vi "MagnetoCaloricSweep_wendel.vi"(9 "Measure for (s)":dbl=5.0, 11 "UseCommandLine":bool=TRUE) -> (1 "Sample temperatur":dbl[](array[numeric]), 2 "Bath Temperature":dbl[](array[numeric]), 3 "Time":u32[](array[numeric]), 4 "XY Graph":cluster{dbl[], dbl[]}[](graph))   [LabVIEW 2019]
uses:
  Instrument_Setup.vi
  Global/Global Variables/Data_Display_global.vi
  Equipment/Lake Shore 372/Lake Shore 372.lvlib
panel:
  in  "Additional LS370":refnum<visa-resource-name>="GPIB0::18::INSTR"
  out "Wait":bool
  in  "Dateipfad (Dialog verwenden)":path
  out "Phi":dbl[](array[numeric])
  out "Field":dbl[](array[numeric])
  out "Indices":i32[](array[numeric])
  out "R2":dbl
  out "R1":dbl
  out "T2":dbl
  out "T1":dbl
  out "Phi":dbl
  out "B":dbl
  in  "StopSkript":bool
  # "current values"
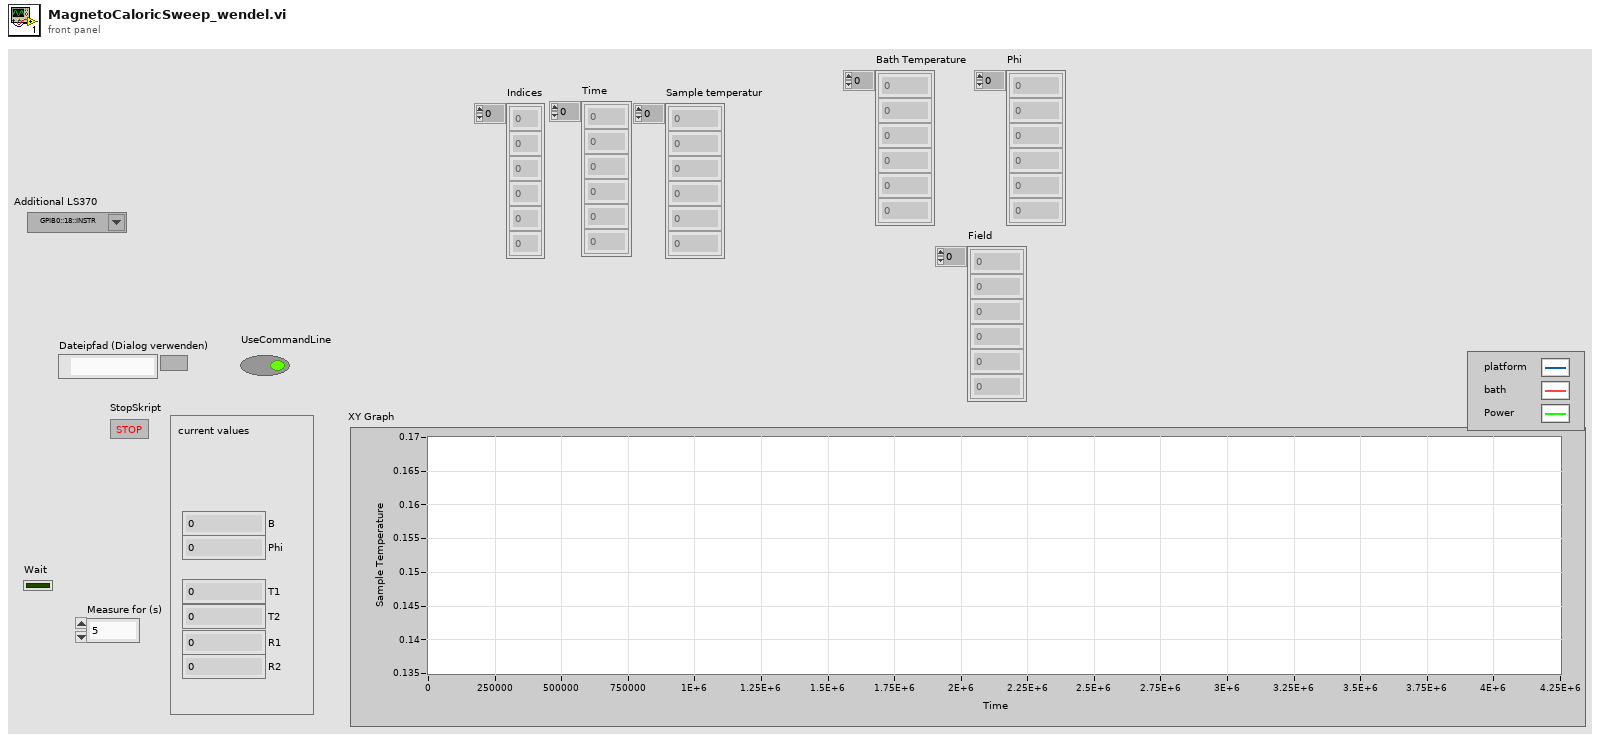
[diagram p1: front panel]
types:
  T1 = enum16{"open", "replace", "create", "open or create", "replace or create", "replace or create with confirmation"}
  T2 = typedef "AMI_cluster.ctl" = cluster{"Y Axis Status":enum16{"", "RAMPING", "HOLDING", "PAUSED", "MANUAL UP", "MANUAL DOWN", "ZEROING CURRENT", "QUENCH DETECTED", "HEATING SWITCH", "AT ZER0", "COOLING SWITCH"}, "Z Axis Status":enum16{"", "RAMPING", "HOLDING", "PAUSED", "MANUAL UP", "MANUAL DOWN", "ZEROING CURRENT", "QUENCH DETECTED", "HEATING SWITCH", "AT ZER0", "COOLING SWITCH"}, "Y-Axis (T)":dbl, "Y-Axis Setpoint (T)":dbl, "Y-Axis Rate (T/min)":dbl, "Z-Axis (T)":dbl, "Z-Axis Setpoint (T)":dbl, "Z-Axis Rate (T/min)":dbl, "B AMI rate (T)":dbl, "AMI Monitor":bool, "AMI Set field rates":bool, "AMI Set field":bool, "Switch Heater Y":bool, "Switch Heater Z":bool, "Switch Heater":bool, "B AMI (T)":dbl, "B AMI Setpoint (T)":dbl, "Phi AMI (Deg) ":dbl, "Phi AMI Setpoint (Deg) ":dbl}
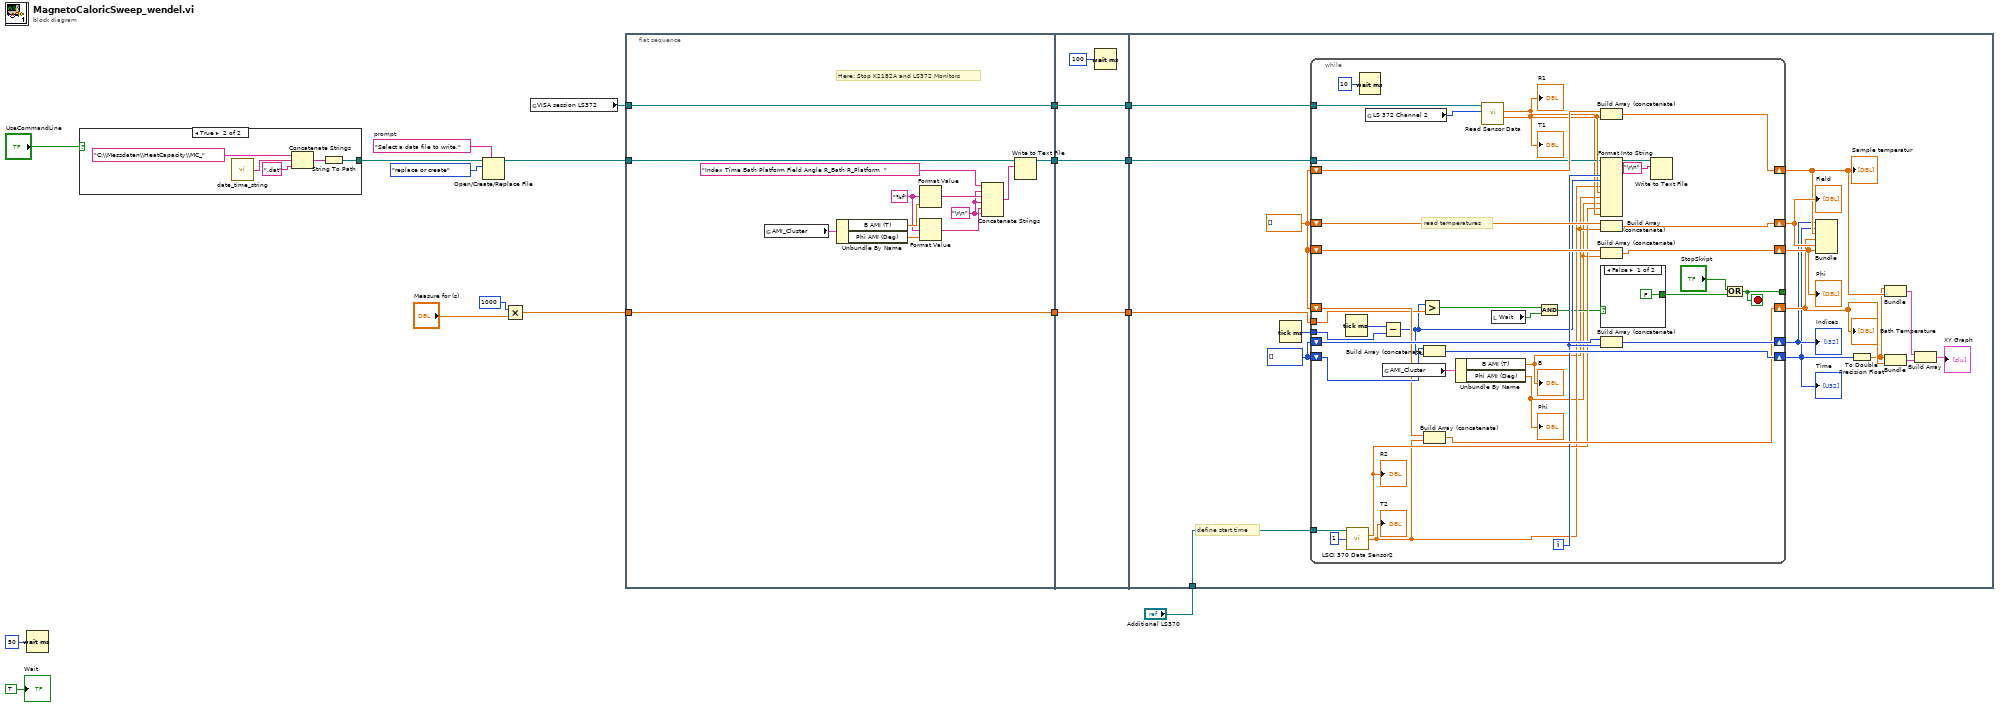
[diagram p0: block diagram]
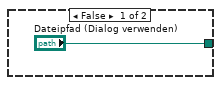
[diagram p2: hidden frame]
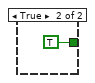
[diagram p3: hidden frame]
diagram:
  w11 = "Select a data file to write."  # prompt
  n1 = Wait (ms)(milliseconds to wait=50) -> ()  [unwired: 1 out]
  n2 = case shown="True" "UseCommandLine" {
    tunnel: ["Dateipfad (Dialog verwenden)" w22] -> w9
    frame False {
    }
    frame True {
      n3 = call "date_time_string.vi"() -> ("date/time string"=w20:string)  [unwired: 1 in]
      n4 = Concatenate Strings("C:\\Messdaten\\HeatCapacity\\MC_", w20, ".dat") -> (w24:string)
      n5 = String To Path(string=w24) -> (path=w22:path)
    }
  }
  n6 = Open/Create/Replace File(file path (use dialog)=w9, prompt=w11, operation (0:open)=T1."replace or create") -> (refnum out=w8:refnum<file>)  [unwired: 3 in, 2 out]
  n7 = Multiply(x=1000, y="Measure for (s)") -> (x*y=w13:dbl)
  n8 = global read "Instrument_Setup.vi" "VISA session LS372"() -> (w17:refnum<visa-resource-name>)
  n9 = flat-sequence {
    tunnel: w13 -> [w36]
    tunnel: w17 -> [w37]
    tunnel: [w37] -> w7
    tunnel: [w36] -> w5
    tunnel: w8 -> [w35]
    tunnel: [w34] -> w3
    tunnel: w7 -> [w41]
    tunnel: [w41] -> w6
    tunnel: w5 -> [w40]
    tunnel: [w40] -> w4
    tunnel: w3 -> [w39]
    tunnel: [w39] -> w2
    tunnel: w6 -> [w58]
    tunnel: w4 -> [w57]
    tunnel: w2 -> [w47]
    tunnel: "Additional LS370" -> [w42]
    frame #0 {
      w27 = "%f"
      w25 = "\r\n"
      # "Here: Stop K2182A and LS372 Monitors"
      n10 = global read "Data_Display_global.vi" "AMI_Cluster"() -> (w31:T2)
      n11 = Unbundle By Name(w31) -> ("B AMI (T)"=w29:dbl, "Phi AMI (Deg)"=w28:dbl)
      n12 = Format Value(format string=w27, value (0)=w29) -> (output string=w30:string)  [unwired: 1 in]
      n13 = Format Value(format string=w27, value (0)=w28) -> (output string=w26:string)  [unwired: 1 in]
      n14 = Concatenate Strings("Index Time Bath Platform Field Angle R_Bath R_Platform  ", w25, w30, w25, w26, w25) -> (w32:string)
      n15 = Write to Text File(file (use dialog)=w35, text=w32) -> (refnum out=w34:refnum<file>)  [unwired: 2 in, 2 out]
    }
    frame #1 {
      n16 = Wait (ms)(milliseconds to wait=100) -> ()  [unwired: 1 out]
    }
    frame #2 {
      w56 = i32[] []
      w55 = dbl[] []
      # "define start time"
      n17 = Tick Count (ms)() -> (millisecond timer value=w46:u32)
      n18 = while {
        shift-right: [w89] -> w45
        shift-left: w56 -> [w90]
        shift-right: [w96] -> w50
        shift-left: w55 -> [w95]
        tunnel: [w75] -> _
        shift-right: [w91] -> w43
        shift-left: w56 -> [w93]
        tunnel: w46 -> [w92]
        tunnel: w58 -> [w67]
        shift-right: [w86] -> w48
        shift-left: w55 -> [w87]
        shift-right: [w84] -> w54
        shift-left: w55 -> [w85]
        shift-right: [w82] -> w53
        shift-left: w55 -> [w83]
        tunnel: w57 -> [w77]
        tunnel: w47 -> [w69]
        tunnel: w42 -> [w63]
        i -> [w81]
        stop <- w75 stop-if-true
        # "read temperatures"
        n19 = Tick Count (ms)() -> (millisecond timer value=w94:u32)
        n20 = call "LSCI 370 Data Sensor2.vi"("VISA session"=w63, "Channel (1)"=1) -> ("Resistance Reading"=w66:dbl, "Kelvin Reading"=w65:dbl)  [unwired: 9 in, 3 out]
        "T2" <- w65
        "R2" <- w66
        n21 = Wait (ms)(milliseconds to wait=10) -> ()  [unwired: 1 out]
        n22 = global read "Instrument_Setup.vi" "LS 372 Channel 2"() -> (w88:u16)
        n23 = Subtract(x=w94, y=w92) -> (x-y=w72:u32)
        n24 = global read "Data_Display_global.vi" "AMI_Cluster"() -> (w62:T2)
        n25 = Greater?(x=w72, y=w77) -> (0:w74:bool)
        n26 = Build Array (concatenate)(w93, w72) -> (w91:u32[])
        n27 = Build Array (concatenate)(w87, w65) -> (w86:dbl[])
        n28 = Unbundle By Name(w62) -> ("B AMI (T)"=w60:dbl, "Phi AMI (Deg)"=w59:dbl)
        "B" <- w60
        "Phi" <- w59
        n29 = call "Read Sensor Data.vi"("Channel (1:1)"=w88, "VISA resource name"=w67) -> ("Kelvin Reading"=w70:dbl, "Resistance Reading"=w68:dbl)  [unwired: 4 in, 4 out]
        "T1" <- w70
        "R1" <- w68
        n30 = local read "Wait"() -> (w73:bool)
        n31 = And(x=w74, y=w73) -> (x .and. y?=w61:bool)
        n32 = Build Array (concatenate)(w95, w70) -> (w96:dbl[])
        n33 = Format Into String(initial string=w69, w81, w72, w65, w70, w60, w59, w66, w68) -> (resulting string=w80:refnum<file>)  [unwired: 2 in, 1 out]
        n34 = Build Array (concatenate)(w85, w60) -> (w84:dbl[])
        n35 = Build Array (concatenate)(w83, w59) -> (w82:dbl[])
        n36 = case shown="False" w61 {
          tunnel: [FALSE TRUE] -> w71
          frame False {
          }
          frame True {
          }
        }
        n37 = Build Array (concatenate)(w90, w81) -> (w89:i32[])
        n38 = Write to Text File(file (use dialog)=w80, text="\r\n") -> ()  [unwired: 2 in, 3 out]
        n39 = Or(x="StopSkript", y=w71) -> (x .or. y?=w75:bool)
      }
      "Sample temperatur" <- w50
      "Time" <- w43
      "Indices" <- w45
      "Bath Temperature" <- w48
      "Field" <- w54
      "Phi" <- w53
      n40 = Bundle(w45, w43, w50, w48, w54, w53) -> ()  [unwired: 1 in, 1 out]
      n41 = To Double Precision Float(number=w43) -> (double precision float=w44:dbl[])
      n42 = Bundle(w44, w50) -> (w52:cluster{dbl[], dbl[]})  [unwired: 1 in]
      n43 = Bundle(w44, w48) -> (w49:cluster{dbl[], dbl[]})  [unwired: 1 in]
      n44 = Build Array(w52, w49) -> (→"XY Graph":cluster{dbl[], dbl[]}[])
    }
  }
  "Wait" <- TRUE
